vi "Read configuration item.vi"(8 "error in (no error)":errorcluster, 10 "configuration item":string, 11 "IConfigDBQueries in":refnum<class "IConfigurationDatabaseQueries.lvclass">) -> (0 "error out":errorcluster, 2 "result":string)   [LabVIEW 2020, in "configuration-database.lvlib" / "IConfigurationDatabaseQueries.lvclass"]
uses:
  IConfigurationDatabaseQueries.lvclass
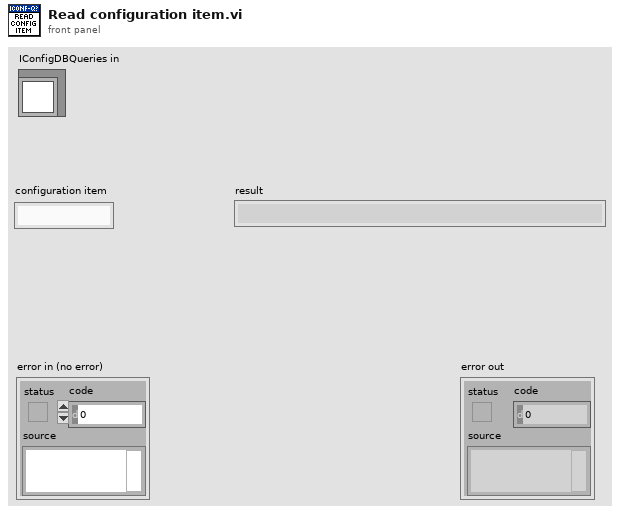
[diagram p1: front panel]
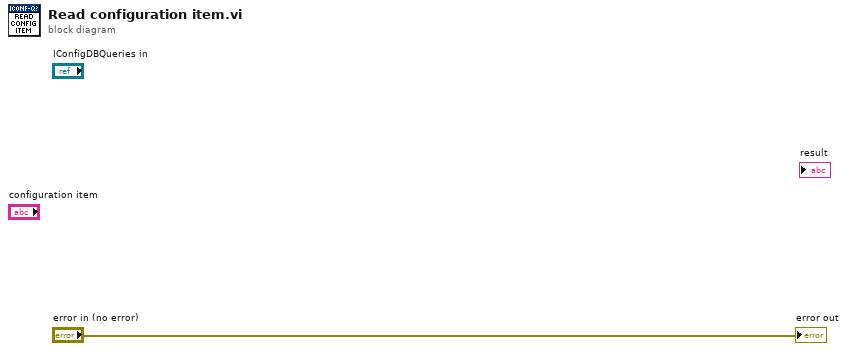
[diagram p0: block diagram]
diagram:
  "error out" <- "error in (no error)"
